vi "Llenado.vi"() -> ()   [LabVIEW 2020]
panel:
  out "Llenado":T1 {"Mezclador" scale=0.0..10.0; "Pintado" scale=0.0..10.0; "Tanque" scale=0.0..100.0; "Llenador" scale=0.0..100.0; "Bote" scale=0.0..100.0}
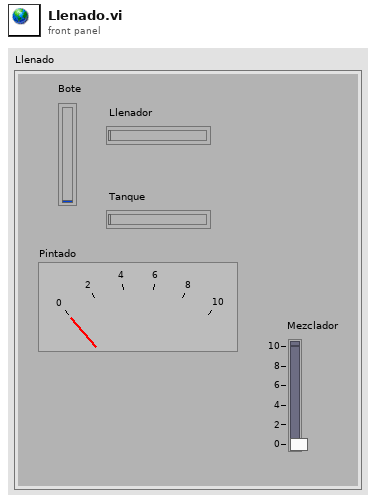
[diagram p1: front panel]
types:
  T1 = cluster{"Bote":u8, "Llenador":u8, "Tanque":u8, "Pintado":dbl, "Mezclador":dbl}
diagram:
